vi "Rinocloud_HTTP_delete.vi"(5 "error in (no error)":errorcluster, 8 "ID":string) -> (0 "error out":errorcluster, 3 "Status":T1={"headers"="", "body"="", "ID"="", "Saved"=TRUE})   [LabVIEW 2013, in "Rinocloud Library.lvlib"]
uses:
  Rinocloud Library.lvlib
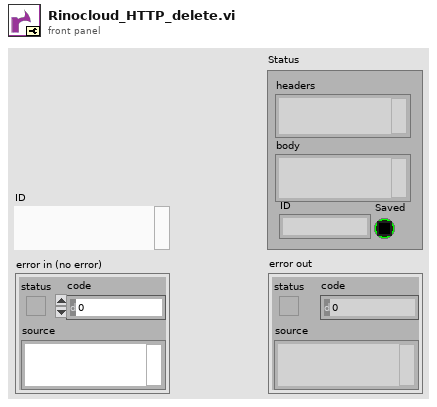
[diagram p1: front panel]
types:
  T1 = cluster{"headers":string, "body":string, "ID":string, "Saved":bool}
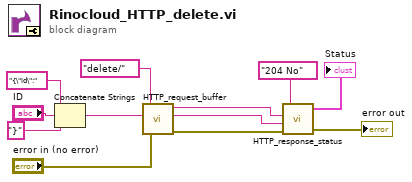
[diagram p0: block diagram]
diagram:
  n1 = Concatenate Strings("{\"id\":" ("string"), "ID", "}" ("string")) -> (w7:string)
  n2 = call "HTTP_request_buffer.vi"("error in (no error)"="error in (no error)", "JSON payload"=w7, "Endpoint"="delete/") -> ("error out"=w9:errorcluster, "body"=w3:string, "headers"=w4:string)  [unwired: 2 in]
  n3 = call "HTTP_response_status.vi"("error in (no error)"=w9, "body"=w3, "headers"=w4, "HTTP status"="204 No") -> ("error out"=→"error out":errorcluster, "Status"=→"Status":T1)  [unwired: 1 in]
